vi "Communication_DataLog.vi"() -> ()   [LabVIEW 2016]
uses:
  Communication/Global communication output.vi
  Communication/Global communication.vi
  Finite State Machine/Sub-VIs/MGCC_FntStaMach_gobal.vi
  <vilib>/Utility/error.llb/Error Cluster From Error Code.vi
  Abnormal Fault State Control/Sub_VIs/Fault_Abnormal_state.vi
  <vilib>/ErrorRing/Error Ring.xnode
panel:
  out "x 3":dbl[][](array[numeric])
  out "Communication all":dbl[](array[numeric])
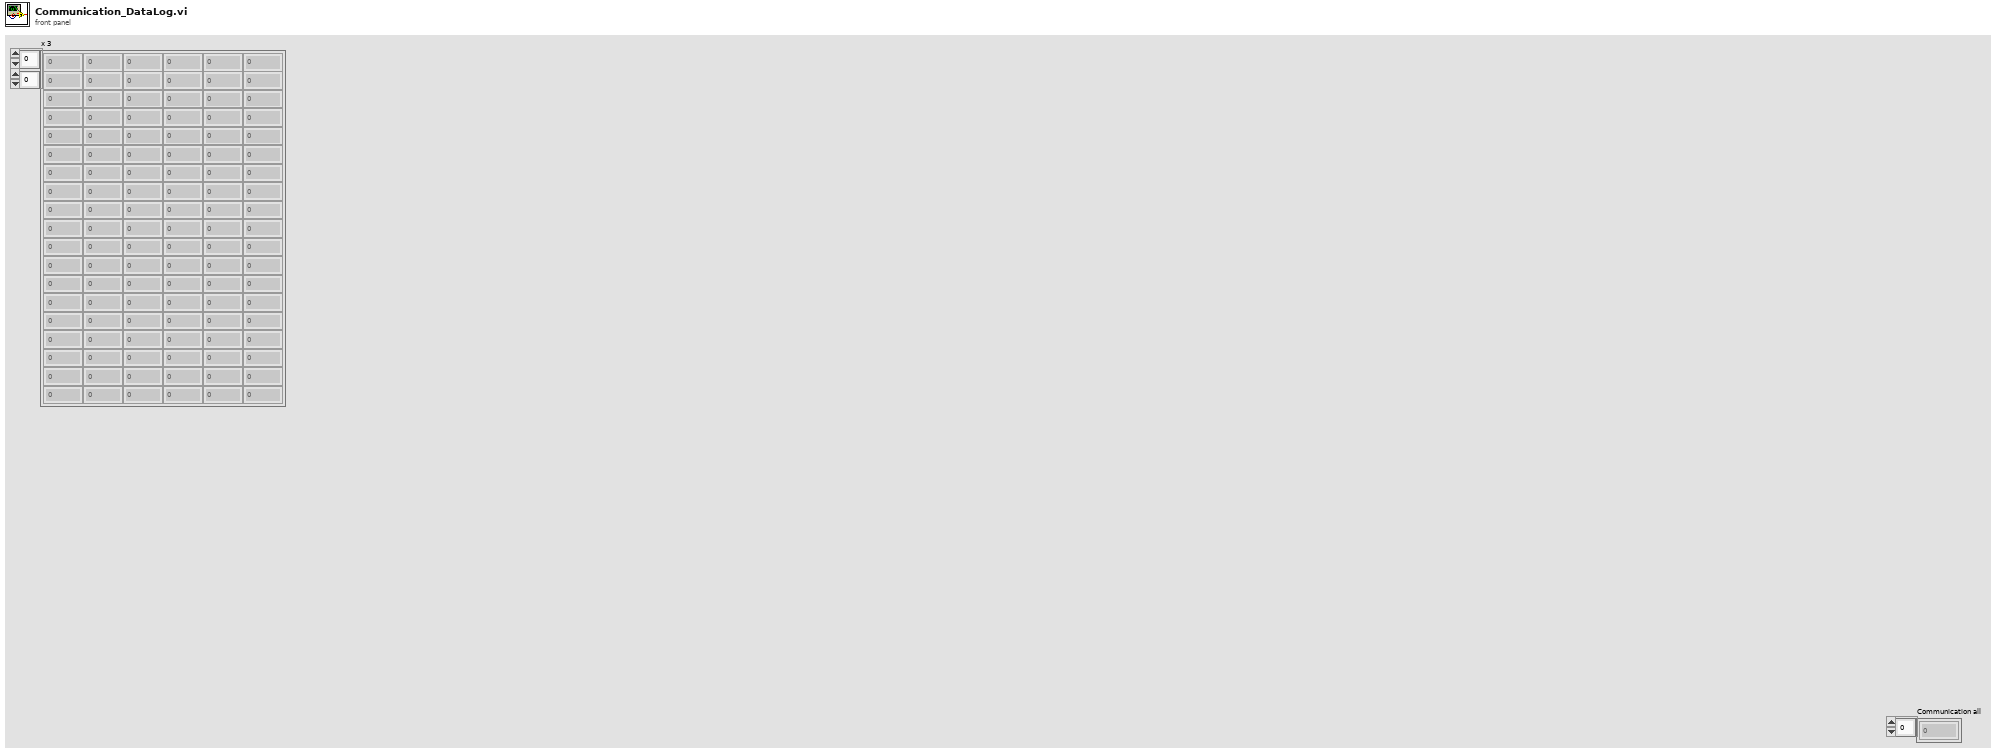
[diagram p1: front panel]
types:
  T1 = enum16{"open", "open or create", "create or replace", "create", "open (read-only)"}
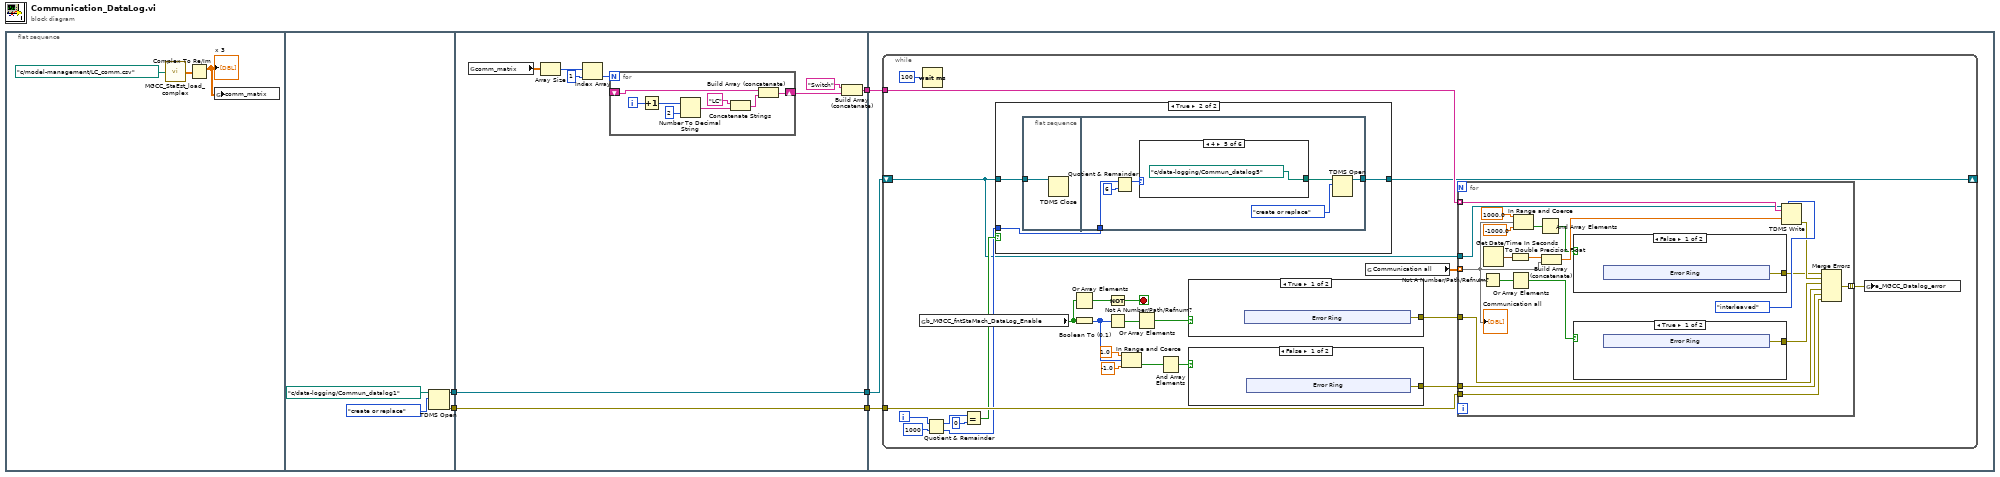
[diagram p0: block diagram]
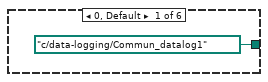
[diagram p3: hidden frame]
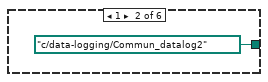
[diagram p4: hidden frame]
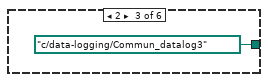
[diagram p5: hidden frame]
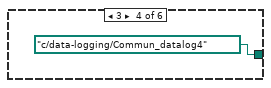
[diagram p6: hidden frame]
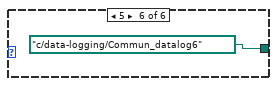
[diagram p7: hidden frame]
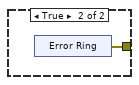
[diagram p8: hidden frame]
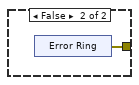
[diagram p9: hidden frame]
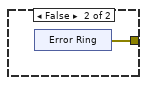
[diagram p10: hidden frame]
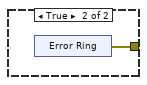
[diagram p11: hidden frame]
diagram:
  n1 = flat-sequence {
    tunnel: [w10] -> w3
    tunnel: [w9] -> w1
    tunnel: [w15] -> w5
    tunnel: [w14] -> w4
    tunnel: w3 -> [w14]
    tunnel: [w13] -> w2
    tunnel: w1 -> [w13]
    tunnel: w5 -> [w32]
    tunnel: w4 -> [w30]
    tunnel: w2 -> [w31]
    frame #0 {
      n2 = call "MGCC_StaEst_load_complex.vi"("file path (dialog if empty)"=path "c:/model-management/LC_comm.csv" ("file path (use dialog)")) -> ("Array 13"=w7:cdb[][])
      n3 = Complex To Re/Im(x + iy=w7) -> (x=w8:dbl[][])  [unwired: 1 out]
      "x 3" <- w8
      n4 = global write "Global communication output.vi" "comm_matrix"(w8) -> ()
    }
    frame #1 {
      n5 = TDMS Open(10:T1."create or replace" ("operation (0:open)"), 11:path "c:/data-logging/Commun_datalog1" ("file path (dialog if empty)")) -> (0:w9:errorcluster, 3:w10:refnum<k34>)  [unwired: 5 in]
    }
    frame #2 {
      n6 = global read "Global communication output.vi" "comm_matrix"() -> (w21:dbl[][])
      n7 = Array Size(array=w21) -> (size(s)=w20:i32[])
      n8 = Index Array(array=w20, index=1) -> (element=w18:i32)
      n9 = for {
        N: w18 -> [_]
        shift-right: [w26] -> w16
        shift-left: _ -> [w27]
        i -> [w23]
        n10 = Increment(x=w23) -> (x+1=w22:i32)
        n11 = Number To Decimal String(number=w22, width (-)=i16 2) -> (decimal integer string=w28:string)
        n12 = Concatenate Strings("LC", w28) -> (w25:string)
        n13 = Build Array (concatenate)(w27, w25) -> (w26:string[])
      }
      n14 = Build Array (concatenate)("Switch", w16) -> (w15:string[])
    }
    frame #3 {
      n15 = while {
        tunnel: w32 -> [w55]
        tunnel: w31 -> [w41]
        shift-right: [w34] -> _
        shift-left: w30 -> [w33]
        i -> [w35]
        stop <- w52 stop-if-true
        n16 = global read "MGCC_FntStaMach_gobal.vi" "b_MGCC_fntStaMach_DataLog_Enable"() -> (w51:bool[])
        n17 = Wait (ms)(milliseconds to wait=u32 100) -> ()  [unwired: 1 out]
        n18 = Quotient & Remainder(x=w35, y=1000) -> (x-y*floor(x/y)=w39:i32, floor(x/y)=w36:i32)
        n19 = Equal?(x=w39, y=0) -> (x = y?=w37:bool)
        n20 = case shown="True" w37 {
          tunnel: w36 -> [_ w61]
          tunnel: w33 -> [w58 w60]
          tunnel: [w58 w59] -> w34
          frame False {
          }
          frame True {
            n21 = flat-sequence {
              tunnel: w60 -> [w62]
              tunnel: w61 -> [w67]
              tunnel: [w63] -> w59
              frame #0 {
                n22 = TDMS Close(11:w62) -> ()  [unwired: 1 in, 2 out]
              }
              frame #1 {
                n23 = Quotient & Remainder(x=w67, y=6) -> (x-y*floor(x/y)=w65:i32)  [unwired: 1 out]
                n24 = case shown="4" w65 {
                  tunnel: [path "c:/data-logging/Commun_datalog1" ("file path (dialog if empty)") path "c:/data-logging/Commun_datalog2" ("file path (dialog if empty)") path "c:/data-logging/Commun_datalog3" ("file path (dialog if empty)") path "c:/data-logging/Commun_datalog4" ("file path (dialog if empty)") path "c:/data-logging/Commun_datalog5" ("file path (dialog if empty)") path "c:/data-logging/Commun_datalog6" ("file path (dialog if empty)")] -> w64
                  frame 0, Default {
                  }
                  frame 1 {
                  }
                  frame 2 {
                  }
                  frame 3 {
                  }
                  frame 4 {
                  }
                  frame 5 {
                  }
                }
                n25 = TDMS Open(10:T1."create or replace" ("operation (0:open)"), 11:w64) -> (3:w63:refnum<k34>)  [unwired: 5 in, 1 out]
              }
            }
          }
        }
        n26 = Or Array Elements(Boolean array=w51) -> (logical OR=w53:bool)
        n27 = Boolean To (0,1)(Boolean=w51) -> (0, 1=w48:i16[])
        n28 = Not(x=w53) -> (.not. x?=w52:bool)
        n29 = Not A Number/Path/Refnum?(number/path/refnum=w48) -> (NaN/Path/Refnum?=w50:bool[])
        n30 = In Range and Coerce(upper limit=1.0, x=w48, lower limit=-1.0 ("upper limit")) -> (In Range?=w45:bool[])  [unwired: 1 out]
        n31 = Or Array Elements(Boolean array=w50) -> (logical OR=w49:bool)
        n32 = And Array Elements(Boolean array=w45) -> (logical AND=w44:bool)
        n33 = case shown="True" w49 {
          tunnel: [w83 w89] -> w43
          frame True {
            n34 = xnode "Error Ring"() -> ("error out"=w83:errorcluster)
          }
          frame False {
            n35 = xnode "Error Ring"() -> ("error out"=w89:errorcluster)
          }
        }
        n36 = case shown="False" w44 {
          tunnel: [w75 w81] -> w42
          frame False {
            n37 = xnode "Error Ring"() -> ("error out"=w75:errorcluster)
          }
          frame True {
            n38 = xnode "Error Ring"() -> ("error out"=w81:errorcluster)
          }
        }
        n39 = global read "Global communication.vi" "Communication all"() -> (w56:dbl[][])
        n40 = for {
          tunnel: w56 -> [w102] mode=indexing
          tunnel: w55 -> [w110] mode=indexing
          tunnel: w33 -> [w108]
          tunnel: [w94] -> w54 mode=indexing
          tunnel: w43 -> [w93]
          tunnel: w42 -> [w92]
          tunnel: w41 -> [w91]
          n41 = Not A Number/Path/Refnum?(number/path/refnum=w102) -> (NaN/Path/Refnum?=w101:bool[])
          n42 = Get Date/Time In Seconds() -> (seconds since 1Jan1904=w107:timestamp)
          n43 = To Double Precision Float(number=w107) -> (double precision float=w106:dbl)
          n44 = Or Array Elements(Boolean array=w101) -> (logical OR=w98:bool)
          n45 = In Range and Coerce(upper limit=1000.0, x=w102, lower limit=-1000.0) -> (In Range?=w100:bool[])  [unwired: 1 out]
          n46 = And Array Elements(Boolean array=w100) -> (logical AND=w99:bool)
          n47 = Build Array (concatenate)(w106, w102) -> (w105:dbl[])
          n48 = case shown="False" w99 {
            tunnel: [w119 w125] -> w96
            frame False {
              n49 = xnode "Error Ring"() -> ("error out"=w119:errorcluster)
            }
            frame True {
              n50 = xnode "Error Ring"() -> ("error out"=w125:errorcluster)
            }
          }
          n51 = case shown="True" w98 {
            tunnel: [w111 w117] -> w95
            frame True {
              n52 = xnode "Error Ring"() -> ("error out"=w111:errorcluster)
            }
            frame False {
              n53 = xnode "Error Ring"() -> ("error out"=w117:errorcluster)
            }
          }
          n54 = TDMS Write(0:w108, 1:enum16{"decimated", "interleaved"}."interleaved" ("data layout (0:decimated)"), 5:w110, 9:w105) -> (15:w97:errorcluster)  [unwired: 2 in, 3 out]
          n55 = Merge Errors(w96, w97, w95, w93, w92, w91) -> (w94:errorcluster)
          "Communication all" <- w102
        }
        n56 = global write "Fault_Abnormal_state.vi" "e_MGCC_Datalog_error"(w54) -> ()
      }
    }
  }
